vi "Disabled.vi"(7 "Robot Mode":T2, 10 "Match Info":T1={"Autonomous Elapsed Seconds"=0.0, "TeleOp Elapsed Seconds"=0.0, "Disabled Elapsed Seconds"=0.0, "Visited Autonomous"=FALSE, "Visited TeleOp"=FALSE, "Visited Disabled"=FALSE, "Autonomous Settings"={"Autonomous Style"=enum."Independent", "VI Refnum"=refnum}}, 11 "Call Context":T3) -> ()   [LabVIEW 2012]
doc: "This VI is called each time a disabled packet is received from the DS. It is often used to prepare for the next robot mode, to calibrate sensors, etc."
uses:
  <vilib>/Rock Robotics/WPI/DriverStation/WPI_DriverStationDerivedRobotMode.ctl
  <vilib>/Rock Robotics/WPI/DriverStation/WPI_DriverStationRobotMode2.ctl
  <vilib>/Rock Robotics/WPI/DriverStation/WPI_DriverStationMatch Info.ctl
  Robot Global Data.vi
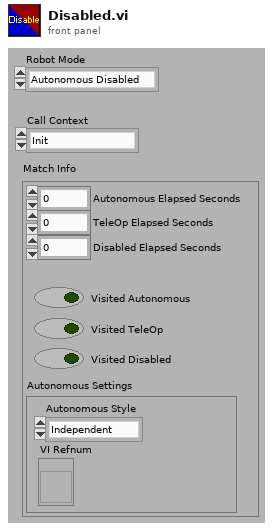
[diagram p1: front panel]
types:
  T1 = typedef "WPI_DriverStationMatch Info.ctl" = cluster{"Autonomous Elapsed Seconds":dbl, "TeleOp Elapsed Seconds":dbl, "Disabled Elapsed Seconds":dbl, "Visited Autonomous":bool, "Visited TeleOp":bool, "Visited Disabled":bool, "Autonomous Settings":cluster{"Autonomous Style":enum16{"Iterative", "Independent"}, "VI Refnum":refnum<vi>}}
  T2 = typedef "WPI_DriverStationRobotMode2.ctl" = enum16{"Autonomous Disabled", "Autonomous Enabled", "Teleop Disabled", "Teleop Enabled", "Timeout", "Finish", "Test Disabled", "Test Enabled"}
  T3 = typedef "WPI_DriverStationDerivedRobotMode.ctl" = enum16{"Init", "Execute", "Stop"}
  T4 = typedef "WPI_MotorControlDeviceRef.ctl" = cluster{"DeviceStatus":errorcluster, "Type":enum16{"PWM", "CAN"}, "PWM":cluster{"Digital Module":T5, "PWM Channel":T6, "DeadBand":T7}, "CAN":cluster{"Device Number":u8, "Control Mode":T8, "Semaphore":T9, "Max Vout":dbl}, "Invert":bool, "TransformRef":T10, "InvTransformRef":T10}
  T5 = typedef "FPGA_TypedefDigitalModule.ctl" = enum16{"Digital Module 1", "Digital Module 2"}
  T6 = typedef "FPGA_DIOPWMChannel.ctl" = enum8{"PWM 1", "PWM 2", "PWM 3", "PWM 4", "PWM 5", "PWM 6", "PWM 7", "PWM 8", "PWM 9", "PWM 10", "Invalid"}
  T7 = typedef "WPI_PWMDeadband.ctl" = cluster{"Name":string, "maxPositivePwm":i32, "minPositivePwm":i32, "centerPwm":i32, "maxNegativePwm":i32, "minNegativePwm":i32, "angularRange":u16}
  T8 = typedef "WPI_CANJaguar_ControlMode.ctl" = enum8{"Percent VBus", "Current", "Speed", "Position", "Voltage"}
  T9 = typedef "Semaphore RefNum" = refnum<k1>
  T10 = typedef "WPI_PWMTransform_ConPane.ctl" = refnum<vi>
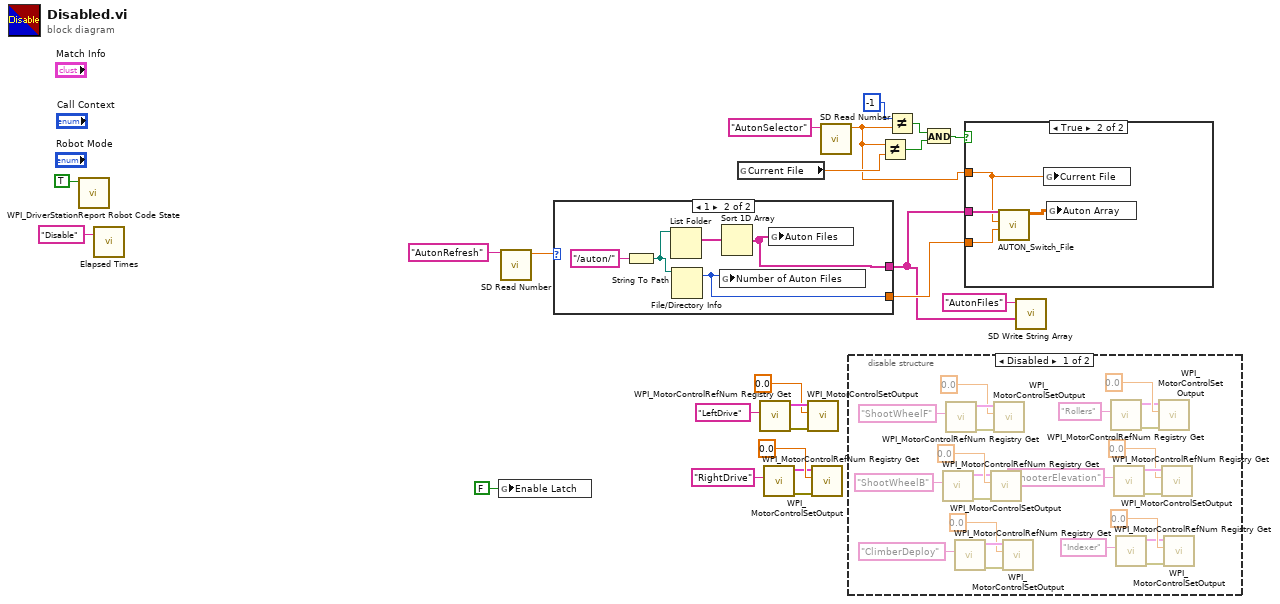
[diagram p0: block diagram]
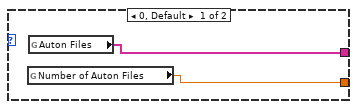
[diagram p4: hidden frame]
diagram:
  n1 = call <vilib>:"WPI_DriverStationReport Robot Code State.vi"("Disabled"=TRUE ("Autonomous")) -> ()  [unwired: 10 in, 1 out]
  n2 = call "Elapsed Times.vi"("Call Name"="Disable") -> ()  [unwired: 2 in, 1 out]
  n3 = global write "Robot Global Data.vi" "Enable Latch"(FALSE ("Enable Latch")) -> ()
  n4 = call <vilib>:"SD Read Number.vi"("Name"="AutonRefresh") -> ("Numeric"=w3:dbl)  [unwired: 8 in, 2 out]
  n5 = case shown="1" w3 {
    tunnel: [w24 w27] -> w13
    tunnel: [w25 w26] -> w8
    frame 0, Default {
      n6 = global read "Robot Global Data.vi" "Number of Auton Files"() -> (w24:dbl)
      n7 = global read "Robot Global Data.vi" "Auton Files"() -> (w25:string[])
    }
    frame 1 {
      n8 = String To Path(string="/auton/") -> (path=w29:path)
      n9 = List Folder(path=w29) -> (filenames=w28:string[])  [unwired: 3 in, 3 out]
      n10 = File/Directory Info(path=w29) -> (size=w27:i64)  [unwired: 1 in, 6 out]
      n11 = global write "Robot Global Data.vi" "Number of Auton Files"(w27) -> ()
      n12 = Sort 1D Array(array=w28) -> (sorted array=w26:string[])
      n13 = global write "Robot Global Data.vi" "Auton Files"(w26) -> ()
    }
  }
  n14 = global read "Robot Global Data.vi" "Current File"() -> (w11:dbl)
  n15 = call <vilib>:"WPI_MotorControlRefNum Registry Get.vi"("refnum name"="LeftDrive") -> ("error out"=w21:errorcluster, "MotorControlDevRef"=w20:T4)  [unwired: 9 in]
  n16 = call <vilib>:"WPI_MotorControlRefNum Registry Get.vi"("refnum name"="RightDrive") -> ("error out"=w14:errorcluster, "MotorControlDevRef"=w15:T4)  [unwired: 9 in]
  n17 = call <vilib>:"WPI_MotorControlSetOutput.vi"("error in (no error)"=w21, "Output"=0.0, "MotorControlDevRef"=w20) -> ()  [unwired: 6 in, 3 out]
  n18 = call <vilib>:"WPI_MotorControlSetOutput.vi"("error in (no error)"=w14, "Output"=0.0, "MotorControlDevRef"=w15) -> ()  [unwired: 6 in, 3 out]
  n19 = call <vilib>:"SD Read Number.vi"("Name"="AutonSelector") -> ("Numeric"=w4:dbl)  [unwired: 8 in, 2 out]
  n20 = disable-structure shown="Disabled" {
    frame Disabled {
      n21 = call <vilib>:"WPI_MotorControlRefNum Registry Get.vi"("refnum name"="ShootWheelB") -> ("error out"=w47:errorcluster, "MotorControlDevRef"=w48:T4)  [unwired: 9 in]
      n22 = call <vilib>:"WPI_MotorControlRefNum Registry Get.vi"("refnum name"="ShootWheelF") -> ("error out"=w54:errorcluster, "MotorControlDevRef"=w53:T4)  [unwired: 9 in]
      n23 = call <vilib>:"WPI_MotorControlRefNum Registry Get.vi"("refnum name"="ClimberDeploy") -> ("error out"=w46:errorcluster, "MotorControlDevRef"=w45:T4)  [unwired: 9 in]
      n24 = call <vilib>:"WPI_MotorControlSetOutput.vi"("error in (no error)"=w47, "Output"=0.0, "MotorControlDevRef"=w48) -> ()  [unwired: 6 in, 3 out]
      n25 = call <vilib>:"WPI_MotorControlSetOutput.vi"("error in (no error)"=w54, "Output"=0.0, "MotorControlDevRef"=w53) -> ()  [unwired: 6 in, 3 out]
      n26 = call <vilib>:"WPI_MotorControlSetOutput.vi"("error in (no error)"=w46, "Output"=0.0, "MotorControlDevRef"=w45) -> ()  [unwired: 6 in, 3 out]
      n27 = call <vilib>:"WPI_MotorControlRefNum Registry Get.vi"("refnum name"="Rollers") -> ("error out"=w39:errorcluster, "MotorControlDevRef"=w40:T4)  [unwired: 9 in]
      n28 = call <vilib>:"WPI_MotorControlRefNum Registry Get.vi"("refnum name"="ShooterElevation") -> ("error out"=w38:errorcluster, "MotorControlDevRef"=w37:T4)  [unwired: 9 in]
      n29 = call <vilib>:"WPI_MotorControlRefNum Registry Get.vi"("refnum name"="Indexer") -> ("error out"=w31:errorcluster, "MotorControlDevRef"=w32:T4)  [unwired: 9 in]
      n30 = call <vilib>:"WPI_MotorControlSetOutput.vi"("error in (no error)"=w39, "Output"=0.0, "MotorControlDevRef"=w40) -> ()  [unwired: 6 in, 3 out]
      n31 = call <vilib>:"WPI_MotorControlSetOutput.vi"("error in (no error)"=w38, "Output"=0.0, "MotorControlDevRef"=w37) -> ()  [unwired: 6 in, 3 out]
      n32 = call <vilib>:"WPI_MotorControlSetOutput.vi"("error in (no error)"=w31, "Output"=0.0, "MotorControlDevRef"=w32) -> ()  [unwired: 6 in, 3 out]
    }
    frame Enabled {
    }
  }
  n33 = Not Equal?(x=w4, y=w11) -> (x != y?=w9:bool)
  n34 = Not Equal?(x=-1, y=w4) -> (x != y?=w10:bool)
  n35 = And(x=w10, y=w9) -> (x .and. y?=w6:bool)
  n36 = case shown="True" w6 {
    tunnel: w8 -> [_ w58]
    tunnel: w13 -> [_ w57]
    tunnel: w4 -> [_ w55]
    frame False {
    }
    frame True {
      n37 = call "AUTON_Switch_File.vi"("Number of Auton Files"=w57, "Auton File"=w55, "Auton Files"=w58) -> ("Auton Array"=w56:dbl[][])  [unwired: 7 in, 1 out]
      n38 = global write "Robot Global Data.vi" "Current File"(w55) -> ()
      n39 = global write "Robot Global Data.vi" "Auton Array"(w56) -> ()
    }
  }
  n40 = call <vilib>:"SD Write String Array.vi"("String Array"=w8, "Name"="AutonFiles") -> ()  [unwired: 8 in, 2 out]
